vi "Remove Backup Config.vi"(8 "error in":errorcluster, 11 "Config File Data In":T1(array[cluster])) -> (0 "error out":errorcluster, 3 "Config Data Out":T1(array[cluster]))   [LabVIEW 2020, in "GUCalibration2.lvlib"]
uses:
  GUCalibration2.lvlib
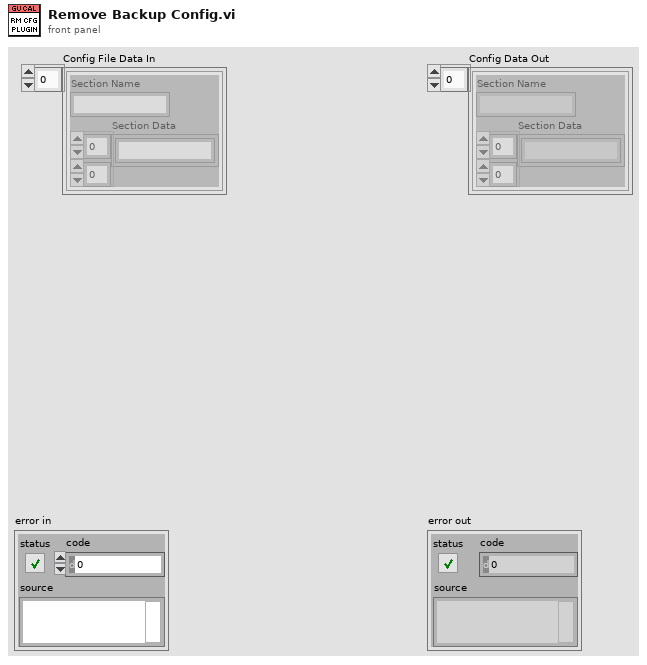
[diagram p1: front panel]
types:
  T1 = cluster{"Section Name":string, "Section Data":string[][]}[]
  T2 = cluster{"Section Name":string, "Section Data":string[][]}
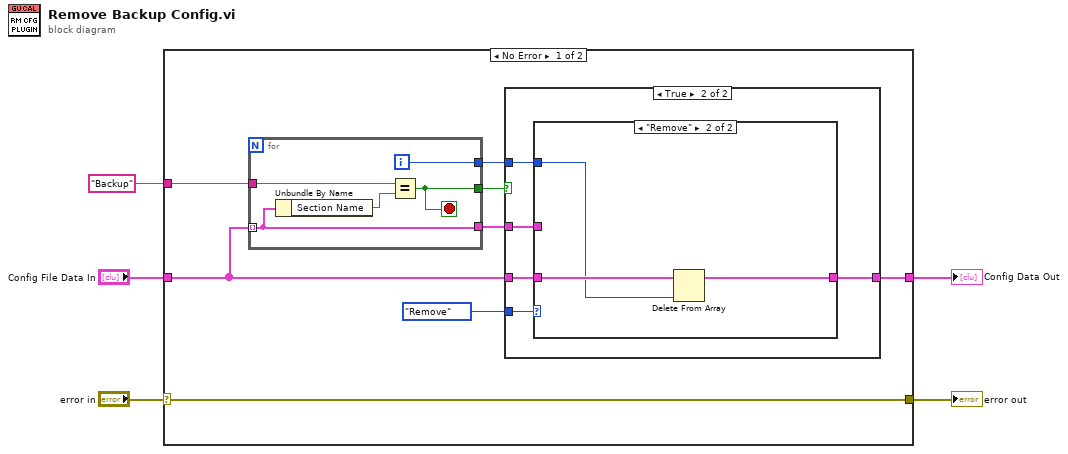
[diagram p0: block diagram]
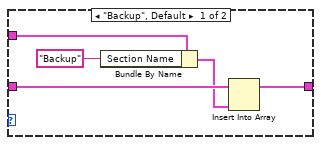
[diagram p3: hidden frame]
diagram:
  n1 = case shown="No Error" "error in" {
    selector: "error in" -> [w8 w34]
    tunnel: "Config File Data In" -> [w11 w33]
    tunnel: "Backup" ("Section Name") -> [w13 _]
    tunnel: [w8 w34] -> w3
    tunnel: [w9 w33] -> w1
    frame No Error {
      n2 = for {
        tunnel: w11 -> [w30] mode=indexing
        tunnel: w13 -> [w32]
        tunnel: [w30] -> w10
        tunnel: [w29] -> w12
        tunnel: [w28] -> w7
        i -> [w28]
        stop <- w29 stop-if-true
        n3 = Unbundle By Name(w30) -> ("Section Name"=w31:string)
        n4 = Equal?(x=w32, y=w31) -> (x = y?=w29:bool)
      }
      n5 = case shown="True" w12 {
        tunnel: w11 -> [w14 w18]
        tunnel: w10 -> [_ w19]
        tunnel: [w14 w17] -> w9
        tunnel: w7 -> [_ w15]
        tunnel: enum16{"Backup", "Remove"}."Remove" ("Action") -> [_ w16]
        frame False {
        }
        frame True {
          n6 = case shown="\"Remove\"" w16 {
            tunnel: w19 -> [w24 _]
            tunnel: w18 -> [w22 w27]
            tunnel: [w21 w25] -> w17
            tunnel: w15 -> [_ w26]
            frame "Backup", Default {
              n7 = Bundle By Name(cluster=w24, "Section Name"="Backup") -> (w20:T2)
              n8 = Insert Into Array(array=w22, new element=w20) -> (w21:T1)  [unwired: 1 in]
            }
            frame "Remove" {
              n9 = Delete From Array(array=w27, index=w26) -> (array with subset deleted=w25:T1)  [unwired: 1 in, 1 out]
            }
          }
        }
      }
    }
    frame Error {
    }
  }
  "error out" <- w3
  "Config Data Out" <- w1
